vi "ADD TASK.vi"(4 "ANALOGICO/DIGITAL":bool, 5 "Adquisicion tiempo":i32, 7 "DAQ BOARD":tag, 8 "error in":errorcluster, 9 "DIGITAL":T1={"Puertos Digital"=[], "Lineas Digital"=[], "Frecuencia Muestreo"=1000, "Puerto/Linea"=FALSE}, 10 "ANALOGICO":T2={"ANALOGICO CANALES"=[], "Numero de muestras"=1000, "Frecuencia de muestreo"=1000}) -> (0 "error out":errorcluster)   [LabVIEW 2020, in "Settings.lvlib"]
doc: "AGREGA EL TASK \n_____\nCreated using Delacor QMH Event Scripter 6.0.0.121."
uses:
  Settings.lvlib
  Acquisition/cluster analogico.ctl
  Acquisition/cluster digital.ctl
  ADD TASK Argument--cluster.ctl
  Acquisition/CONTROLS.lvlib
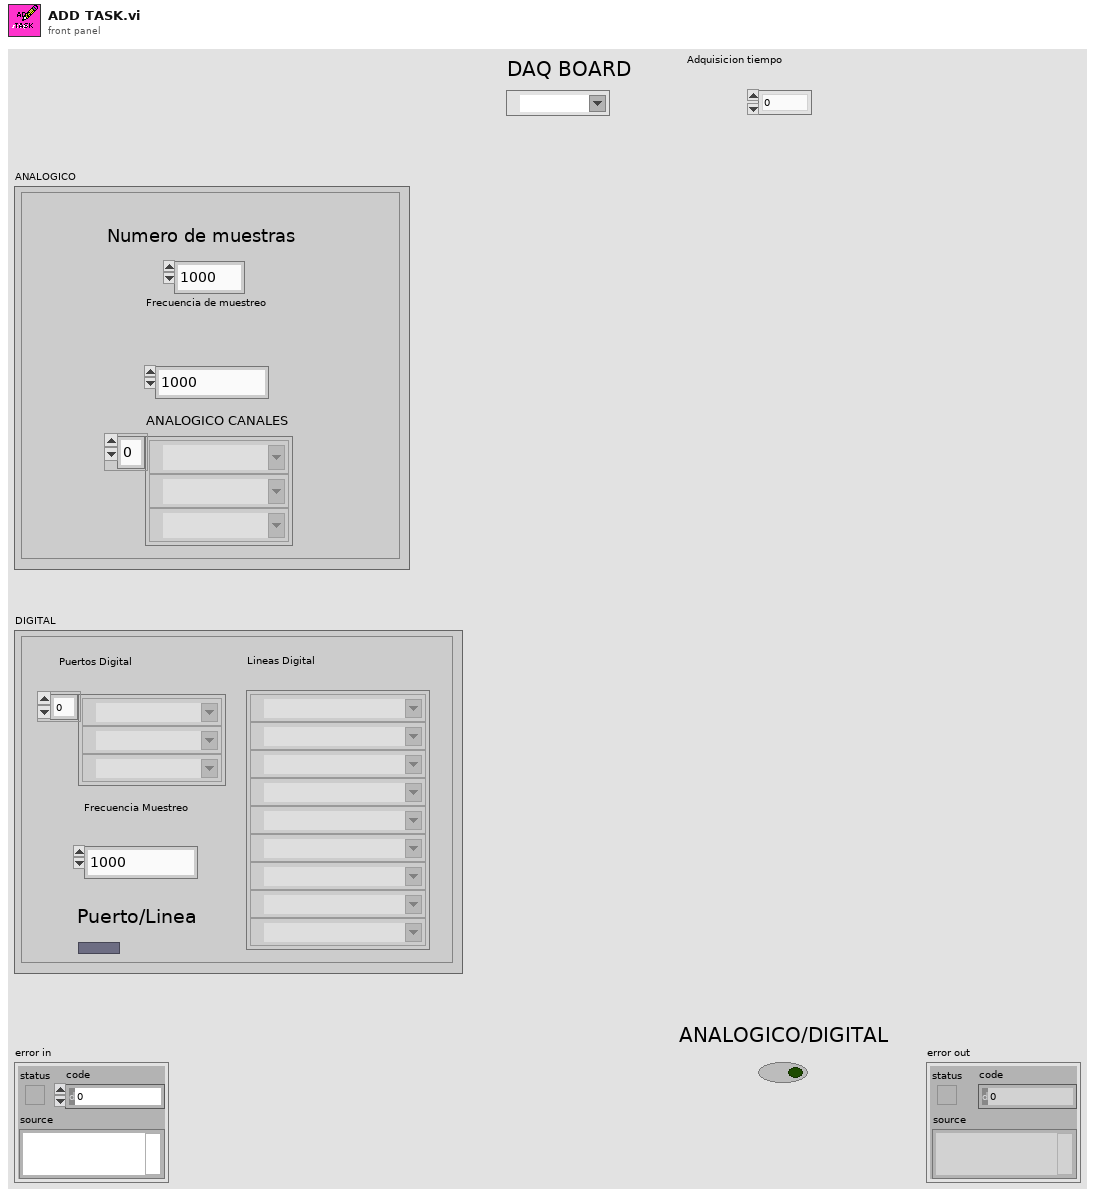
[diagram p1: front panel]
types:
  T1 = typedef "Acquisition.lvlib/CONTROLS.lvlib/cluster digital.ctl" = cluster{"Puertos Digital":tag[], "Lineas Digital":tag[], "Frecuencia Muestreo":u32, "Puerto/Linea":bool}
  T2 = typedef "Acquisition.lvlib/CONTROLS.lvlib/cluster analogico.ctl" = cluster{"ANALOGICO CANALES":tag[], "Numero de muestras":u32, "Frecuencia de muestreo":u32}
  T3 = typedef "Settings.lvlib/ADD TASK Argument--cluster.ctl" = cluster{"ANALOGICO":T2, "DIGITAL":T1, "DAQ BOARD":tag, "Adquisicion tiempo":i32, "ANALOGICO/DIGITAL":bool}
  T4 = typedef "Settings.lvlib/Request Events--cluster.ctl" = cluster{"Stop Module":refnum<user-event>, "Show Panel":refnum<user-event>, "Hide Panel":refnum<user-event>, "Get Module Execution Status":refnum<user-event>, "Show Diagram":refnum<user-event>, "ADD TASK":refnum<user-event>, "Erase all":refnum<user-event>}
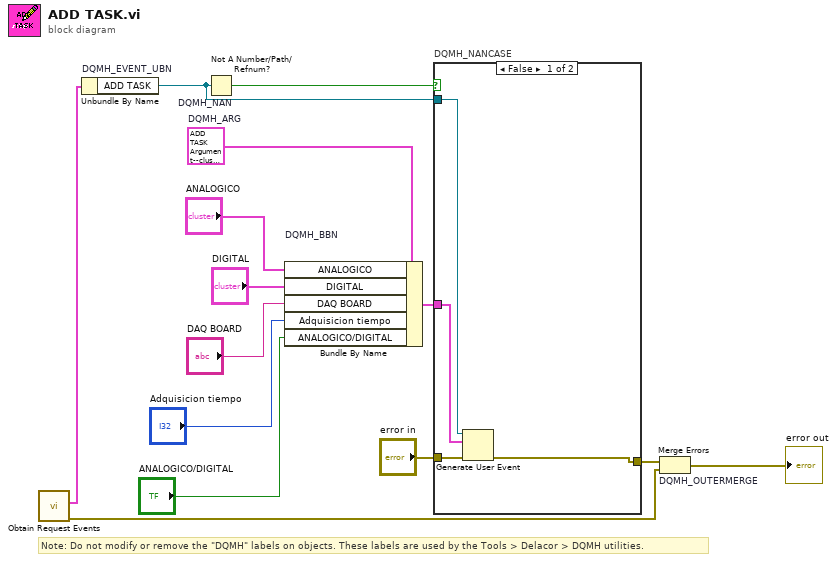
[diagram p0: block diagram]
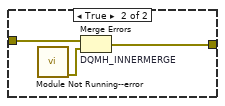
[diagram p2: hidden frame]
diagram:
  w8 = T3 {"ANALOGICO"={"ANALOGICO CANALES"=[], "Numero de muestras"=1000, "Frecuencia de muestreo"=1000}, "DIGITAL"={"Puertos Digital"=[], "Lineas Digital"=[], "Frecuencia Muestreo"=1000, "Puerto/Linea"=FALSE}, "DAQ BOARD"="", "Adquisicion tiempo"=0, "ANALOGICO/DIGITAL"=FALSE}  # DQMH_ARG
  # "Note: Do not modify or remove the \"DQMH\" labels on objects. These labels are used by the Tools > Delacor > DQMH utilities."
  n1 = call "Obtain Request Events.vi"() -> ("error out"=w2:errorcluster, "Settings Request Events"=w1:T4)  [unwired: 10 in]
  n2 = Unbundle By Name "DQMH_EVENT_UBN"(w1) -> ("ADD TASK"=w10:refnum<user-event>)
  n3 = Not A Number/Path/Refnum? "DQMH_NAN"(number/path/refnum=w10) -> (NaN/Path/Refnum?=w11:bool)
  n4 = Bundle By Name "DQMH_BBN"(cluster=w8, "ANALOGICO"="ANALOGICO", "DIGITAL"="DIGITAL", "DAQ BOARD"="DAQ BOARD", "Adquisicion tiempo"="Adquisicion tiempo", "ANALOGICO/DIGITAL"="ANALOGICO/DIGITAL") -> (w12:T3)
  n5 = case "DQMH_NANCASE" shown="False" w11 {
    tunnel: "error in" -> [w18 w21]
    tunnel: [w17 w20] -> w9
    tunnel: w10 -> [w16 _]
    tunnel: w12 -> [w15 _]
    frame False {
      n6 = Generate User Event(user event=w16, event data cluster=w15, error in=w18) -> (error out=w17:errorcluster)  [unwired: 1 in, 1 out]
    }
    frame True {
      n7 = call "Module Not Running--error.vi"() -> ("error out"=w19:errorcluster)  [unwired: 11 in]
      n8 = Merge Errors "DQMH_INNERMERGE"(w21, w19) -> (w20:errorcluster)
    }
  }
  n9 = Merge Errors "DQMH_OUTERMERGE"(w9, w2) -> (→"error out":errorcluster)
